vi "Measure DC offset in TDMS.vi"(4 "Waveform dt":dbl, 5 "Waveform length":i64, 6 "Offset duration":dbl format="%0.2f", 7 "Waveform start":i64, 8 "Error In":errorcluster, 9 "channel name in":string, 10 "group name in":string, 11 "tdms file":refnum<k34>) -> (0 "Error Out":errorcluster, 2 "Offset":dbl format="%0.2f", 3 "tdms file out":refnum<k34>)   [LabVIEW 2021]
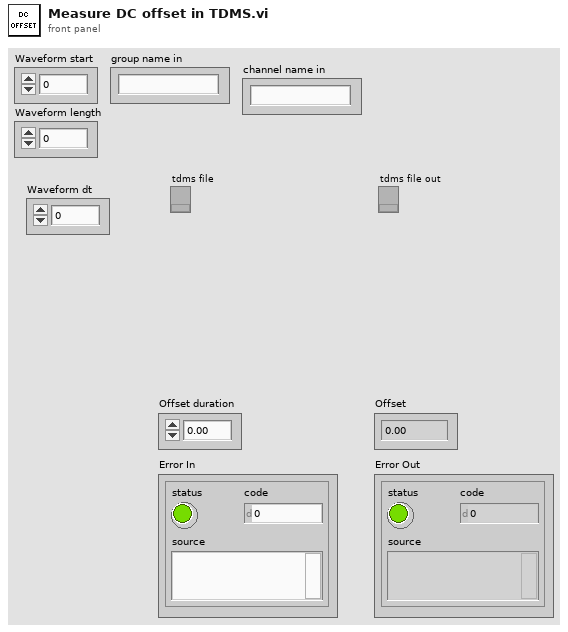
[diagram p1: front panel]
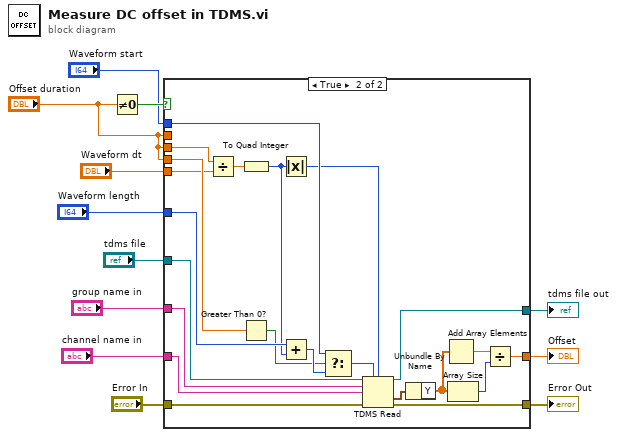
[diagram p0: block diagram]
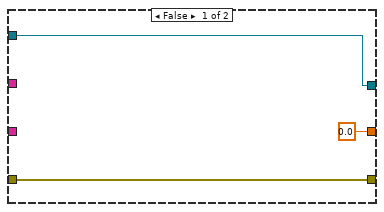
[diagram p2: hidden frame]
diagram:
  n1 = Not Equal To 0?(x="Offset duration") -> (x != 0?=w12:bool)
  n2 = case shown="True" w12 {
    tunnel: "Offset duration" -> [_ _]
    tunnel: [w13 w30] -> w11
    tunnel: [0.0 w34] -> w10
    tunnel: "group name in" -> [_ w33]
    tunnel: "channel name in" -> [_ w32]
    tunnel: "Error In" -> [w13 w31]
    tunnel: "Waveform start" -> [_ w29]
    tunnel: "Waveform length" -> [_ w27]
    tunnel: "Offset duration" -> [_ w23]
    tunnel: "Waveform dt" -> [_ w21]
    tunnel: "Offset duration" -> [_ w20]
    tunnel: "tdms file" -> [w14 w18]
    tunnel: [w14 w17] -> w1
    frame False {
    }
    frame True {
      n3 = Divide(x=w20, y=w21) -> (x/y=w19:dbl)
      n4 = To Quad Integer(1:w19) -> (0:w24:i64)
      n5 = Greater Than 0?(x=w23) -> (x > 0?=w22:bool)
      n6 = Absolute Value(x=w24) -> (abs(x)=w25:i64)
      n7 = Add(x=w27, y=w24) -> (x+y=w26:i64)
      n8 = Select(t=w29, s=w22, f=w26) -> (s? t:f=w28:i64)
      n9 = TDMS Read(0:w18, 1:w28, 2:w25, 5:w33, 7:w32, 11:w31) -> (4:w17:refnum<k34>, 10:w16:waveform(dbl), 15:w30:errorcluster)  [unwired: 2 in, 3 out]
      n10 = Unbundle By Name(w16) -> ("Y"=w36:dbl[])
      n11 = Add Array Elements(numeric array=w36) -> (sum=w35:dbl)
      n12 = Array Size(array=w36) -> (size(s)=w37:i32)
      n13 = Divide(x=w35, y=w37) -> (x/y=w34:dbl)
    }
  }
  "Error Out" <- w11
  "Offset" <- w10
  "tdms file out" <- w1
